vi "Wait For Viewer.vi"(8 "error in (no error)":errorcluster, 9 "timeout ms (wait forever: -1)":i32, 11 "Data Server Thread in":refnum<class "Data Server Thread.lvclass">) -> (0 "error out":errorcluster, 1 "timed out?":bool, 2 "viewer":T1, 3 "Data Server Thread out":refnum<class "Data Server Thread.lvclass">)   [LabVIEW 2017, in "DSF Core.lvlib" / "Data Server Thread.lvclass"]
uses:
  Data Server Thread.lvclass
  Viewer Data.ctl
  Buffer/Buffer.lvclass
  Data Server Thread.lvclass/Data Server Thread.ctl
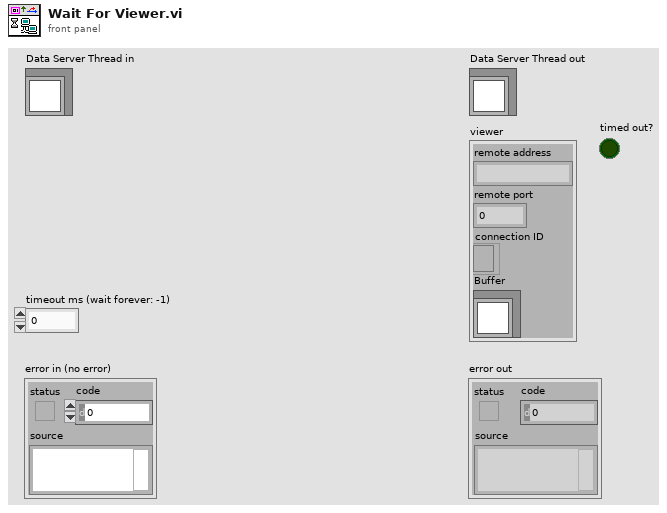
[diagram p1: front panel]
types:
  T1 = typedef "DSF Core.lvlib/Data Server Thread.lvclass/Viewer Data.ctl" = cluster{"remote address":string, "remote port":u16, "connection ID":refnum<k5>, "Buffer":refnum<class "Buffer.lvclass">}
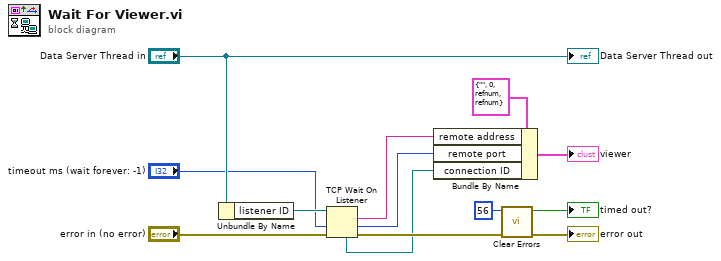
[diagram p0: block diagram]
diagram:
  n1 = Unbundle By Name("Data Server Thread in") -> ("listener ID"=w9:refnum<k5>)
  n2 = TCP Wait On Listener(8:"error in (no error)", 9:"timeout ms (wait forever: -1)", 11:w9) -> (0:w12:errorcluster, 1:w3:u16, 2:w4:string, 4:w2:refnum<k5>)  [unwired: 1 in, 1 out]
  n3 = Bundle By Name(cluster=T1 {"remote address"="", "remote port"=0, "connection ID"=refnum, "Buffer"=refnum} ("viewer"), "remote address"=w4, "remote port"=w3, "connection ID"=w2) -> (→"viewer":T1)
  n4 = call <vilib>:"Clear Errors.vi"("error in (no error)"=w12, "specific error code to clear (0: all)"=56) -> ("error out"=→"error out":errorcluster, "specific error cleared?"=→"timed out?":bool)  [unwired: 4 in]
  "Data Server Thread out" <- "Data Server Thread in"
